vi "Face_Detection_Read_Iamges_by_Paths.vi"(0 "Dataset Path (Images)":path, 1 "Max Sample count":i32=300, 7 "Img Height":i32, 9 "Img Width":i32, 11 "error in (no error)":errorcluster, 12 "Img Type":enum16{"Grayscale", "RGB"}(ring)) -> (4 "NN_DataSet(In3D_OutBBox)":T1={"Inputs Ref."=variant(refnum<data-value> refnum), "Dataset_Size"=0, "Dims_In"={"C"=0, "H"=0, "W"=0}, "Outputs Refs"=refnum, "No of Classes "=0, "Labels"=[], "File Paths"=[]}, 15 "error out":errorcluster)   [LabVIEW 2020]
uses:
  <vilib>/Ngene/Deep Learning Toolkit/Toolkit/NN_Data/API/DataSet/DataSet_Types/NN_DataSet(In3D_OutBBox).ctl
  <vilib>/Ngene/Deep Learning Toolkit/Toolkit/NN_Data/API/NN_Dims(C,H,W).ctl
  <vilib>/Ngene/Deep Learning Toolkit/Toolkit/NN_Data/Controls/DataRef_Types/1D/NN_Data_ref(1D_BBox).ctl
  <vilib>/Ngene/Deep Learning Toolkit/Toolkit/NN_Data/API/Data/Detection_Types/NN_Image_Annotations.ctl
  <vilib>/Ngene/Deep Learning Toolkit/Toolkit/NN_Data/API/Data/Detection_Types/NN_BBox_Annotation.ctl
  <vilib>/Ngene/Deep Learning Toolkit/Toolkit/NN_Data/API/Data/Detection_Types/NN_BBox.ctl
  <vilib>/Analysis/1siggen.llb/Riffle Array (I32).vi
  <vilib>/vision/NI_Vision_Development_Module.lvlib
  <vilib>/Ngene/Deep Learning Toolkit/Toolkit/Deep_Learning_Toolkit_by_Ngene.lvlib
  <vilib>/Analysis/NI_AALBase.lvlib
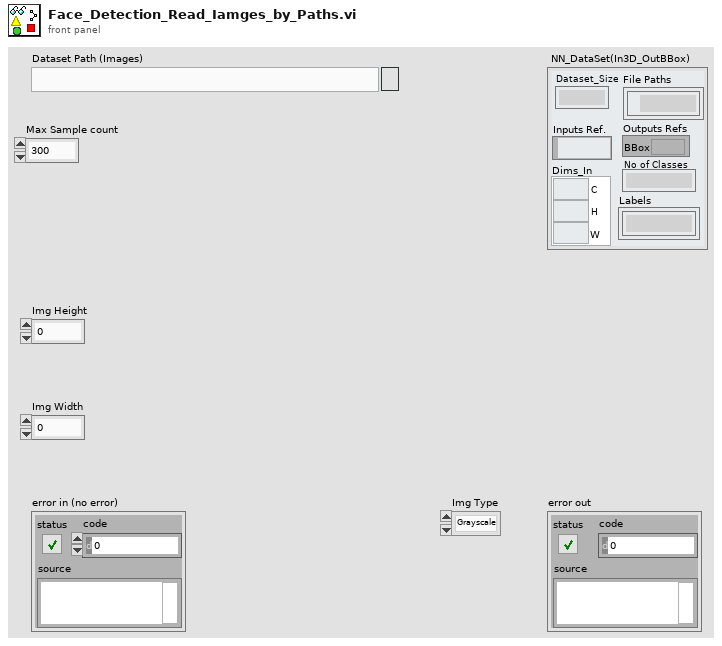
[diagram p1: front panel]
types:
  T1 = typedef "Deep_Learning_Toolkit_by_Ngene.lvlib/NN_DataSet(In3D_OutBBox).ctl" = cluster{"Inputs Ref.":variant, "Dataset_Size":i32, "Dims_In":T2, "Outputs Refs":T3, "No of Classes ":i32, "Labels":string[], "File Paths":path[]}
  T2 = typedef "Deep_Learning_Toolkit_by_Ngene.lvlib/NN_Dims(C,H,W).ctl" = cluster{"C":i32, "H":i32, "W":i32}
  T3 = typedef "Deep_Learning_Toolkit_by_Ngene.lvlib/NN_Data_ref(1D_BBox).ctl" = refnum<data-value>
  T4 = typedef "Image Type" = u32
  T5 = typedef "IMAQ Image.ctl" = refnum<image>
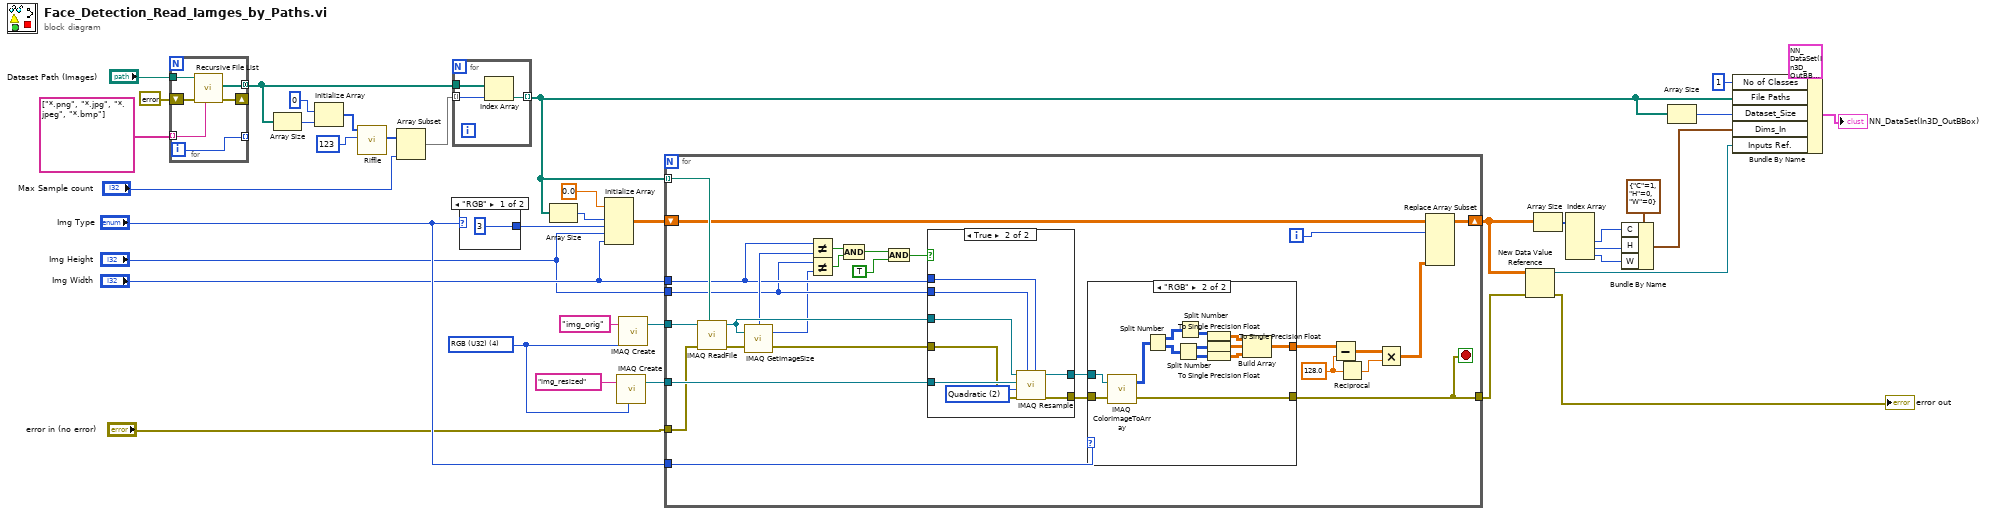
[diagram p0: block diagram]
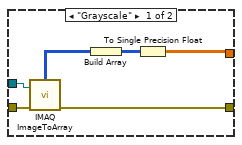
[diagram p2: hidden frame]
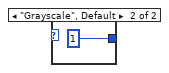
[diagram p4: hidden frame]
diagram:
  w30 = T4 4 items=["Grayscale (U8)", "Grayscale (I16)", "Grayscale (SGL)", "Complex (CSG)", "RGB (U32)", "HSL (U32)", "RGB (U64)", "Grayscale (U16)"] ("Image Type")
  n1 = for {
    tunnel: "Dataset Path (Images)" -> [w45]
    tunnel: string[] ["*.png", "*.jpg", "*.jpeg", "*.bmp"] ("pattern") -> [w44] mode=indexing
    tunnel: [w43] -> w5 mode=concatenating
    shift-right: [w41] -> _
    shift-left: errorcluster {"status"=FALSE, "code"=0, "source"=""} ("error out") -> [w42]
    tunnel: [w40] -> _ mode=indexing
    i -> [w40]
    n2 = call <vilib>:"Recursive File List.vi"("pattern"=w44, "error in (no error)"=w42, "Folder Path"=w45) -> ("error out"=w41:errorcluster, "All Files in Dir"=w43:path[])  [unwired: 4 in, 3 out]
  }
  n3 = Array Size(array=w5) -> (size(s)=w4:i32)
  n4 = Initialize Array(0 ("seed"), w4) -> (w2:i32[])
  n5 = call-poly <vilib>:"Riffle.vi"("seed"=123, "X"=w2) -> ("Riffled Index"=w1:i32[])  [unwired: 7 in, 2 out]
  n6 = Array Subset(array=w1, length="Max Sample count") -> (w8:i32[])  [unwired: 1 in]
  n7 = for {
    tunnel: [w48] -> w10 mode=indexing
    tunnel: w5 -> [w47]
    tunnel: w8 -> [w46] mode=indexing
    n8 = Index Array(array=w47, index=w46) -> (element=w48:path)
  }
  n9 = case shown="\"RGB\"" "Img Type" {
    tunnel: [3 1] -> w20
    frame "RGB" {
    }
    frame "Grayscale", Default {
    }
  }
  n10 = Array Size(array=w10) -> (size(s)=w37:i32)
  n11 = Initialize Array(sgl 0.0 ("element"), w37, w20, "Img Height", "Img Width") -> (w24:sgl[][][][])
  n12 = call "IMAQ Create"("Image Name"="img_resized", "Image Type"=w30) -> ("New Image"=w23:T5)  [unwired: 3 in, 1 out]
  n13 = call "IMAQ Create"("Image Name"="img_orig", "Image Type"=w30) -> ("New Image"=w18:T5)  [unwired: 3 in, 1 out]
  n14 = for {
    tunnel: w18 -> [w78]
    tunnel: w23 -> [w76]
    tunnel: w10 -> [w74] mode=indexing
    shift-right: [w72] -> w16
    shift-left: w24 -> [w73]
    tunnel: "Img Height" -> [w64]
    tunnel: "Img Width" -> [w65]
    tunnel: "Img Type" -> [w58]
    tunnel: "error in (no error)" -> [w70]
    tunnel: [w59] -> w29
    i -> [w71]
    stop <- w59 stop-if-true
    w54 = sgl 128.0 ("element")
    n15 = call "IMAQ ReadFile"("File Path"=w74, "error in (no error)"=w70, "Image"=w78) -> ("error out"=w69:errorcluster, "Image Out"=w67:T5)  [unwired: 4 in, 3 out]
    n16 = call "IMAQ GetImageSize"("Image"=w67, "error in (no error)"=w69) -> ("Y Resolution"=w63:i32, "X Resolution"=w66:i32, "error out"=w68:errorcluster)  [unwired: 2 in]
    n17 = Not Equal?(x=w65, y=w66) -> (x != y?=w62:bool)
    n18 = Not Equal?(x=w64, y=w63) -> (x != y?=w61:bool)
    n19 = Compound Arithmetic op=AND(w62, w61) -> (w60:bool)
    n20 = And(x=w60, y=TRUE ("value")) -> (x .and. y?=w57:bool)
    n21 = case shown="True" w57 {
      tunnel: w67 -> [w99 w107]
      tunnel: [w99 w106] -> w77
      tunnel: w76 -> [_ w105]
      tunnel: w68 -> [w98 w104]
      tunnel: [w98 w103] -> w75
      tunnel: w64 -> [_ w102]
      tunnel: w65 -> [_ w101]
      frame False {
      }
      frame True {
        w100 = u32 2 items=["Zero Order", "Bi-Linear", "Quadratic", "Cubic Spline"] ("Interpolation Type")
        n22 = call "IMAQ Resample"("X Resolution"=w101, "Y Resolution"=w102, "error in (no error)"=w104, "Interpolation Type"=w100, "Image Dst"=w105, "Image Src"=w107) -> ("error out"=w103:errorcluster, "Image Dst Out"=w106:T5)  [unwired: 4 in]
      }
    }
    n23 = case shown="\"RGB\"" w58 {
      tunnel: w77 -> [w84 w97]
      tunnel: w75 -> [w83 w96]
      tunnel: [w81 w94] -> w59
      tunnel: [w79 w85] -> w53
      frame "Grayscale" {
        n24 = call "IMAQ ImageToArray"("error in (no error)"=w83, "Image"=w84) -> ("error out"=w81:errorcluster, "Image Pixels (U8)"=w82:u8[][])  [unwired: 2 in, 3 out]
        n25 = Build Array(w82) -> (w80:u8[][][])
        n26 = To Single Precision Float(number=w80) -> (single precision float=w79:sgl[][][])
      }
      frame "RGB" {
        n27 = call "IMAQ ColorImageToArray"("Image"=w97, "error in (no error)"=w96) -> ("Image Pixels (U32)"=w95:u32[][], "error out"=w94:errorcluster)  [unwired: 2 in, 1 out]
        n28 = Split Number(x=w95) -> (hi(x)=w92:u16[][], lo(x)=w93:u16[][])
        n29 = Split Number(x=w93) -> (hi(x)=w90:u8[][], lo(x)=w89:u8[][])
        n30 = Split Number(x=w92) -> (lo(x)=w91:u8[][])  [unwired: 1 out]
        n31 = To Single Precision Float(number=w91) -> (single precision float=w88:sgl[][])
        n32 = To Single Precision Float(number=w90) -> (single precision float=w87:sgl[][])
        n33 = To Single Precision Float(number=w89) -> (single precision float=w86:sgl[][])
        n34 = Build Array(w88, w87, w86) -> (w85:sgl[][][])
      }
    }
    n35 = Subtract(x=w53, y=w54) -> (x-y=w55:sgl[][][])
    n36 = Reciprocal(x=w54) -> (1/x=w51:sgl)
    n37 = Multiply(x=w55, y=w51) -> (x*y=w52:sgl[][][])
    n38 = Replace Array Subset(array=w73, new element=w52, index (dim 0)=w71) -> (w72:sgl[][][][])  [unwired: 3 in]
  }
  n39 = New Data Value Reference(data value=w16, error in=w29) -> (data value reference=w28:refnum<data-value>, error out=→"error out":errorcluster)
  n40 = Array Size(array=w16) -> (size(s)=w32:i32[])
  n41 = Index Array(array=w32) -> (element #2=w33:i32, element #3=w34:i32, element #4=w35:i32)  [unwired: 4 in, 1 out]
  n42 = Bundle By Name(cluster=T2 {"C"=1, "H"=0, "W"=0} ("Dims"), "C"=w33, "H"=w34, "W"=w35) -> (w36:T2)
  n43 = Array Size(array=w10) -> (size(s)=w11:i32)
  n44 = Bundle By Name(cluster=T1 {"Inputs Ref."=variant(refnum<data-value> refnum), "Dataset_Size"=0, "Dims_In"={"C"=0, "H"=0, "W"=0}, "Outputs Refs"=refnum, "No of Classes "=0, "Labels"=["large", "small"], "File Paths"=[]} ("Train DataSet"), "No of Classes"=1, "File Paths"=w10, "Dataset_Size"=w11, "Dims_In"=w36, "Inputs Ref."=w28) -> (→"NN_DataSet(In3D_OutBBox)":T1)
